vi "dvp Vi Get Contrast.vi"(10 "pContrast":i32, 11 "handle":u32) -> (2 "pContrast out":i32, 3 "function return":u32(ring))   [LabVIEW 2018, in "LabViewDVPCamera.lvlib"]
doc: "LabviewDvp2Api dvpStatus dvpViGetContrast(dvpHandle handle, dvpInt32 *pContrast);"
uses:
  LabViewDVPCamera.lvlib
  LabViewDVPCamera/LabViewDVPCamera.dll
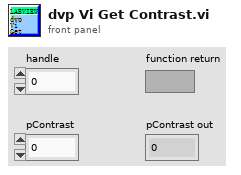
[diagram p1: front panel]
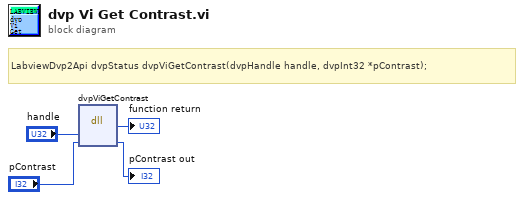
[diagram p0: block diagram]
diagram:
  # "LabviewDvp2Api dvpStatus dvpViGetContrast(dvpHandle handle, dvpInt32 *pContrast);"
  n1 = dll-call lib="C:/Program Files (x86)/DVP2 Labview cn 64/Sample/LabViewDVPCamera/LabViewDVPCamera.*" fn="dvpViGetContrast"("handle"="handle", "pContrast"="pContrast") -> (→"function return":u32, "pContrast"=→"pContrast out":i32)  [unwired: 4 in, 2 out]
